vi "angulardistribution.vi"() -> ()   [LabVIEW 2024]
panel:
  out "THL":dbl
  out "2-14-25":i32
  out "1-13-25":i32
  out "23-11-25":i32
  out "12-24-25":i32
  in  "THL Discriminator 12":i32(slide) min=-250 max=0 step=5 scale=0.0..-250.0
  out "Seconds":i32
  out "10-22-25":i32
  out "9-21-25":i32
  out "8-20-25":i32
  out "7-19-25":i32
  out "6-18-25":i32
  out "5-17-25":i32
  out "4-16-25":i32
  out "3-15-25":i32
  in  "STOP":bool
  in  "START":bool
  in  "EXIT":bool
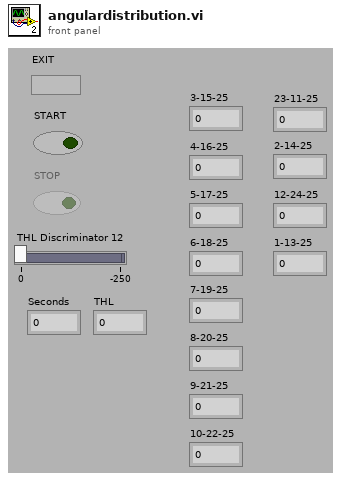
[diagram p1: front panel]
types:
  T1 = enum16{"Connect", "Set A", "Set B", "Set C", "Set D", "Set E", "Set F", "Set G", "Set H", "Get AND", "Read Counter", "Clear Counter"}
  T2 = enum16{"Connect", "Get IN", "Write Threshold", "Write Hysteresis", "Write Stretch"}
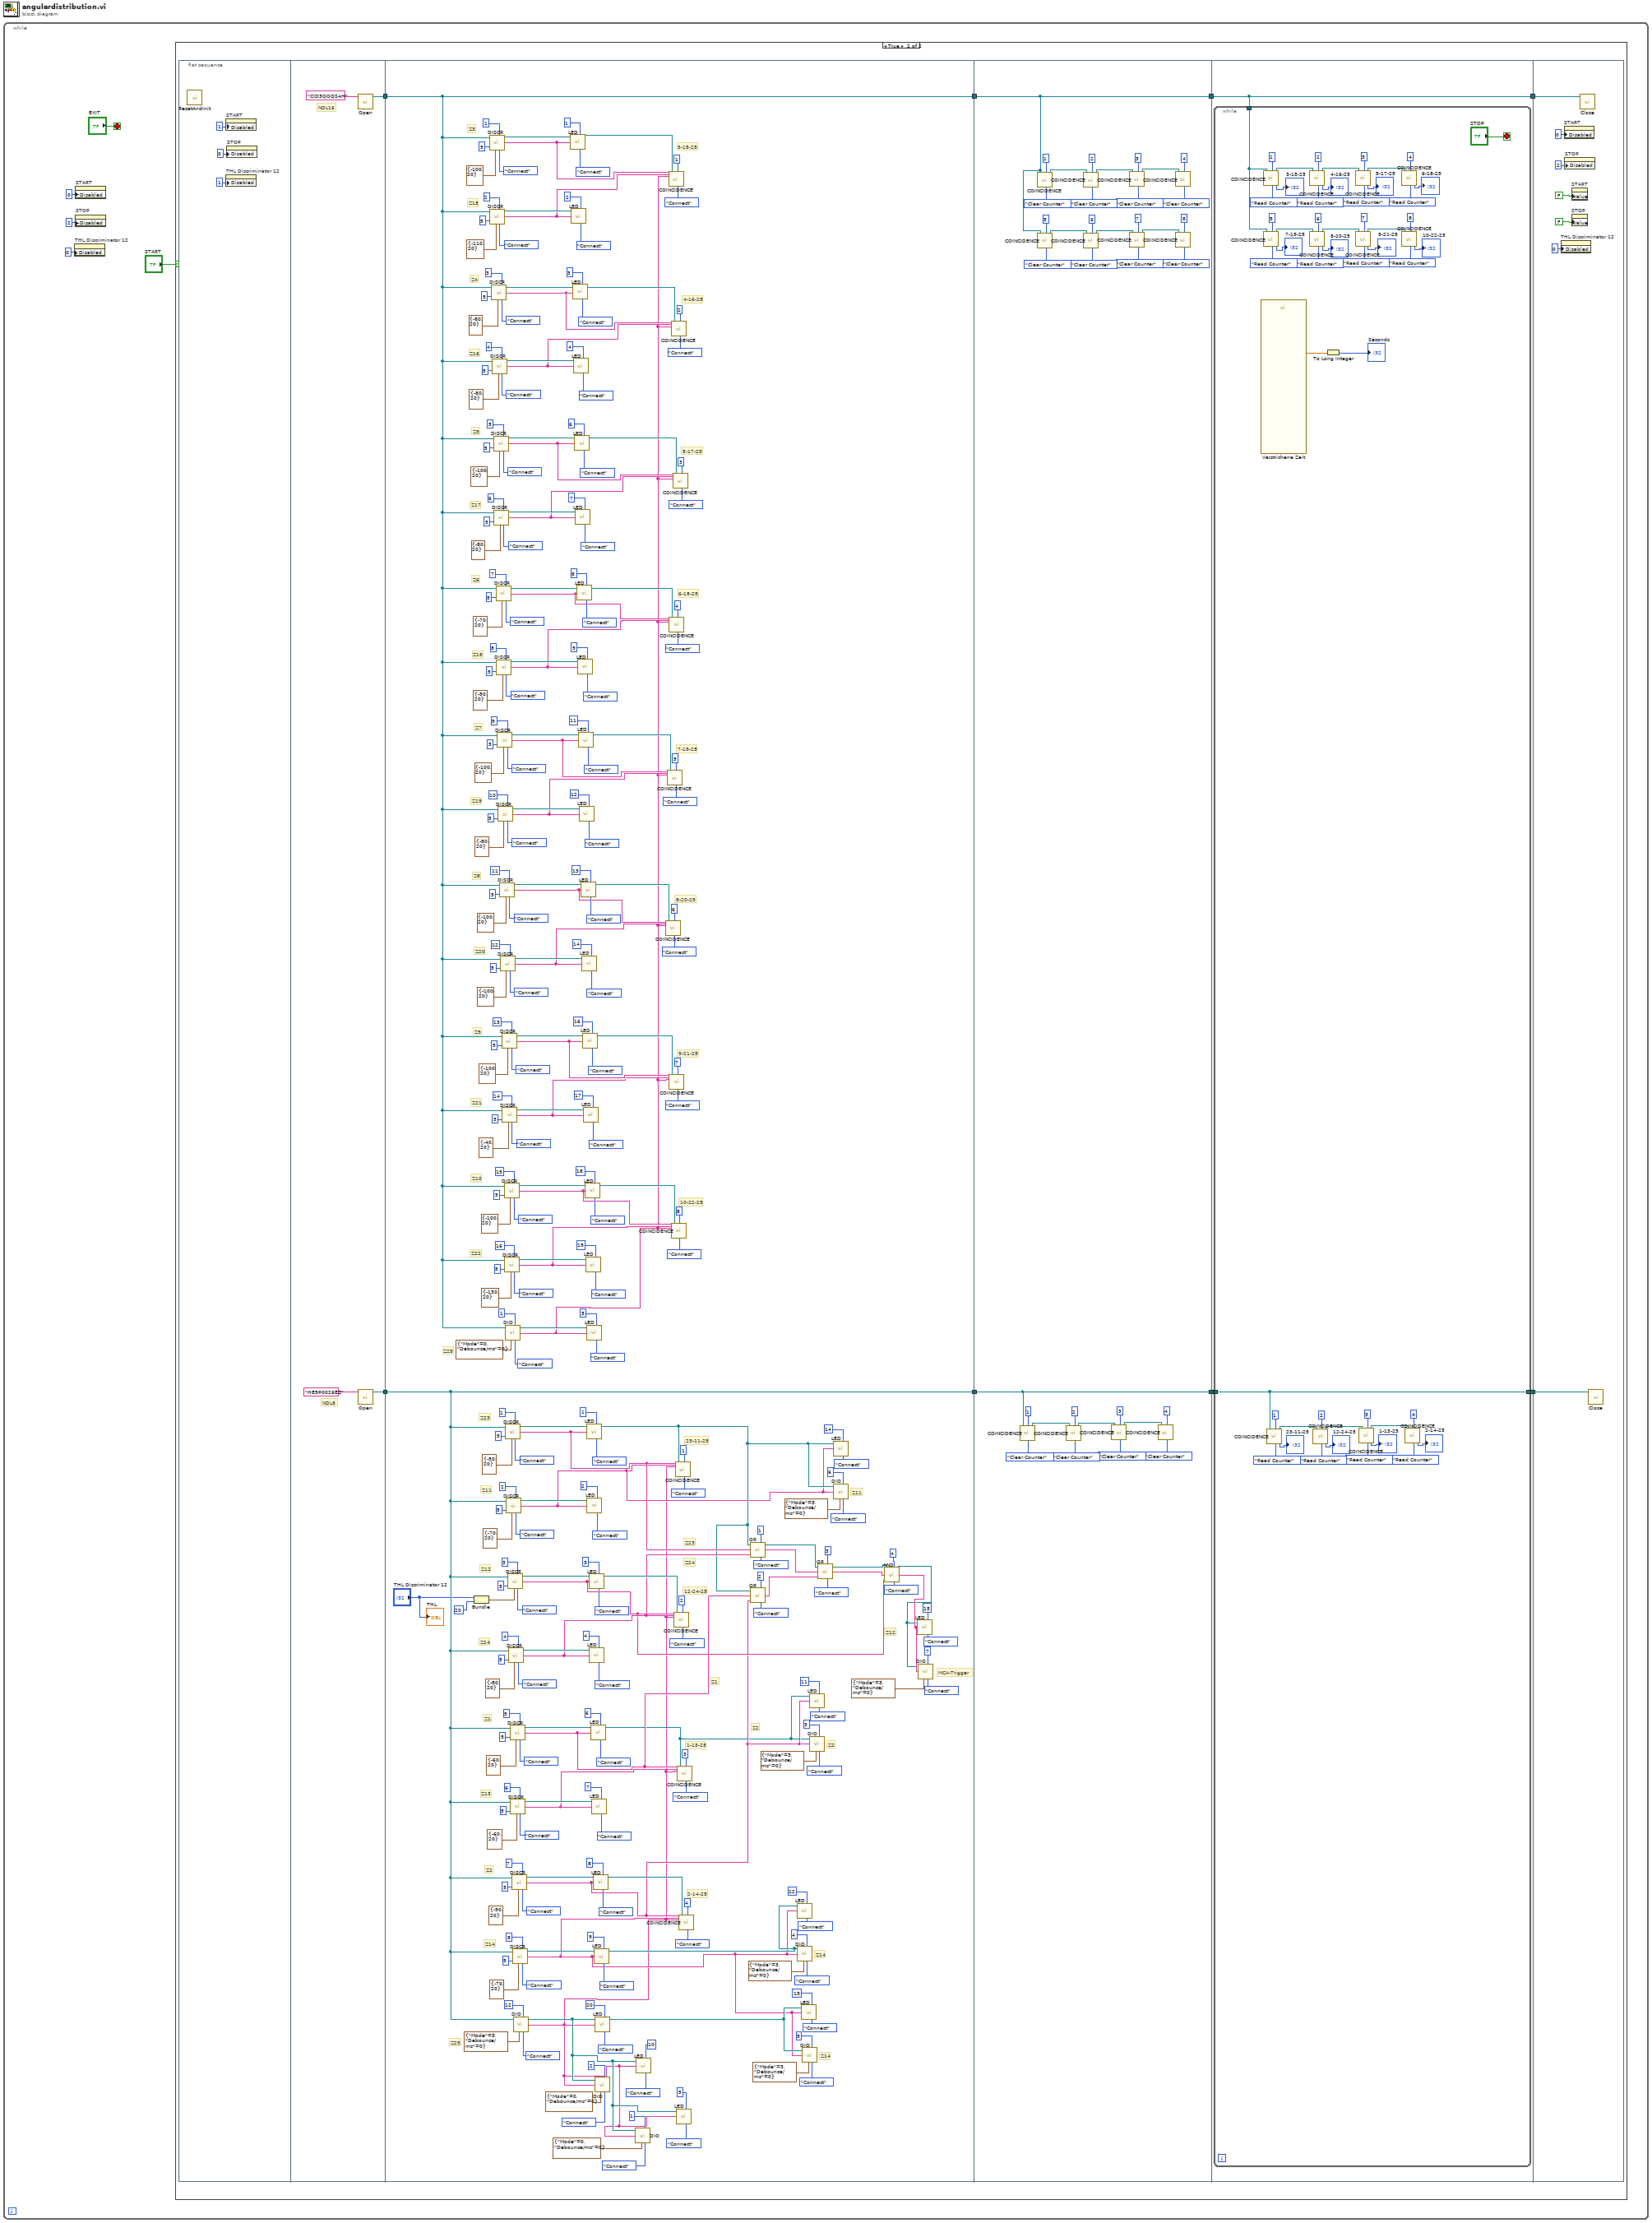
[diagram p0: block diagram]
diagram:
  n1 = while {
    stop <- "EXIT" stop-if-true
    n2 = property on="THL Discriminator 12" class="Schieber (strikt)"("Disabled"=u8 0 ("Deaktiviert")) -> ()  [unwired: 2 in, 2 out]
    n3 = property on="START" class="Bool. (strikt)"("Disabled"=u8 0 ("Deaktiviert")) -> ()  [unwired: 2 in, 2 out]
    n4 = property on="STOP" class="Bool. (strikt)"("Disabled"=u8 2 ("Deaktiviert")) -> ()  [unwired: 2 in, 2 out]
    n5 = case shown="True" "START" {
      frame False {
      }
      frame True {
        n6 = flat-sequence {
          tunnel: [w20] -> w13
          tunnel: [w17] -> w6
          tunnel: w13 -> [w31]
          tunnel: [w31] -> w12
          tunnel: [w92] -> w7
          tunnel: w6 -> [w92]
          tunnel: w12 -> [w331]
          tunnel: [w331] -> w11
          tunnel: [w319] -> w8
          tunnel: w7 -> [w319]
          tunnel: w11 -> [w356]
          tunnel: [w356] -> w10
          tunnel: [w355] -> w9
          tunnel: w8 -> [w354]
          tunnel: w10 -> [w411]
          tunnel: w9 -> [w407]
          frame #0 {
            n7 = call <userlib>:"ResetAndInit.vi"() -> ()  [unwired: 1 out]
            n8 = property on="START" class="Bool. (strikt)"("Disabled"=u8 1 ("Deaktiviert")) -> ()  [unwired: 2 in, 2 out]
            n9 = property on="THL Discriminator 12" class="Schieber (strikt)"("Disabled"=u8 1 ("Deaktiviert")) -> ()  [unwired: 2 in, 2 out]
            n10 = property on="STOP" class="Bool. (strikt)"("Disabled"=u8 0 ("Deaktiviert")) -> ()  [unwired: 2 in, 2 out]
          }
          frame #1 {
            # "NDL8"
            # "NDL16"
            n11 = call <userlib>:"Open.vi"("USB_LogicBox"="CID3QOQS4H") -> ("USB Out"=w20:refnum<visa-resource-name>)  [unwired: 1 in, 7 out]
            n12 = call <userlib>:"Open.vi"("USB_LogicBox"="HE5P0026EZ") -> ("USB Out"=w17:refnum<visa-resource-name>)  [unwired: 1 in, 7 out]
          }
          frame #2 {
            # "Z11"
            # "Z14"
            # "Z14"
            # "Z2"
            # "Z12"
            # "Z2"
            # "Z24"
            # "Z23"
            # "Z1"
            # "MCA-Trigger"
            # "2-14-25"
            # "1-13-25"
            # "12-24-25"
            # "23-11-25"
            # "Z25"
            # "Z14"
            # "Z2"
            # "Z13"
            # "Z1"
            # "Z24"
            # "Z12"
            # "Z11"
            # "Z23"
            # "10-22-25"
            # "9-21-25"
            # "8-20-25"
            # "7-19-25"
            # "6-18-25"
            # "5-17-25"
            # "4-16-25"
            # "3-15-25"
            # "Z25"
            # "Z22"
            # "Z10"
            # "Z21"
            # "Z9"
            # "Z20"
            # "Z8"
            # "Z19"
            # "Z7"
            # "Z18"
            # "Z6"
            # "Z17"
            # "Z5"
            # "Z16"
            # "Z4"
            # "Z15"
            # "Z3"
            n13 = Bundle("THL Discriminator 12"="THL Discriminator 12", 20) -> (w70:cluster{"THL Discriminator 12":i32, i32})  [unwired: 1 out]
            n14 = call <userlib>:"DISCR.vi"("USB In"=w31, "Stretch/10ns"=u8 5, "Params"=cluster{"Threshold/mV":i16, "Hysteresis/mV":u16} {"Threshold/mV"=-100, "Hysteresis/mV"=20}, "DISCR#"=u8 1, "Function"=T2."Connect") -> ("USB Out"=w314:refnum<visa-resource-name>, "DISCR"=w38:string)  [unwired: 3 out]
            n15 = call <userlib>:"DISCR.vi"("USB In"=w31, "Stretch/10ns"=u8 5, "Params"=cluster{"Threshold/mV":i16, "Hysteresis/mV":u16} {"Threshold/mV"=-110, "Hysteresis/mV"=20}, "DISCR#"=u8 2, "Function"=T2."Connect") -> ("USB Out"=w307:refnum<visa-resource-name>, "DISCR"=w37:string)  [unwired: 3 out]
            n16 = call <userlib>:"DISCR.vi"("USB In"=w31, "Stretch/10ns"=u8 5, "Params"=cluster{"Threshold/mV":i16, "Hysteresis/mV":u16} {"Threshold/mV"=-80, "Hysteresis/mV"=20}, "DISCR#"=u8 3, "Function"=T2."Connect") -> ("USB Out"=w300:refnum<visa-resource-name>, "DISCR"=w196:string)  [unwired: 3 out]
            n17 = call <userlib>:"DISCR.vi"("USB In"=w31, "Stretch/10ns"=u8 5, "Params"=cluster{"Threshold/mV":i16, "Hysteresis/mV":u16} {"Threshold/mV"=-80, "Hysteresis/mV"=20}, "DISCR#"=u8 4, "Function"=T2."Connect") -> ("USB Out"=w293:refnum<visa-resource-name>, "DISCR"=w194:string)  [unwired: 3 out]
            n18 = call <userlib>:"DISCR.vi"("USB In"=w31, "Stretch/10ns"=u8 5, "Params"=cluster{"Threshold/mV":i16, "Hysteresis/mV":u16} {"Threshold/mV"=-100, "Hysteresis/mV"=20}, "DISCR#"=u8 5, "Function"=T2."Connect") -> ("USB Out"=w286:refnum<visa-resource-name>, "DISCR"=w180:string)  [unwired: 3 out]
            n19 = call <userlib>:"DISCR.vi"("USB In"=w31, "Stretch/10ns"=u8 5, "Params"=cluster{"Threshold/mV":i16, "Hysteresis/mV":u16} {"Threshold/mV"=-80, "Hysteresis/mV"=20}, "DISCR#"=u8 6, "Function"=T2."Connect") -> ("USB Out"=w279:refnum<visa-resource-name>, "DISCR"=w179:string)  [unwired: 3 out]
            n20 = call <userlib>:"DISCR.vi"("USB In"=w31, "Stretch/10ns"=u8 5, "Params"=cluster{"Threshold/mV":i16, "Hysteresis/mV":u16} {"Threshold/mV"=-70, "Hysteresis/mV"=20}, "DISCR#"=u8 7, "Function"=T2."Connect") -> ("USB Out"=w272:refnum<visa-resource-name>, "DISCR"=w177:string)  [unwired: 3 out]
            n21 = call <userlib>:"DISCR.vi"("USB In"=w31, "Stretch/10ns"=u8 5, "Params"=cluster{"Threshold/mV":i16, "Hysteresis/mV":u16} {"Threshold/mV"=-50, "Hysteresis/mV"=20}, "DISCR#"=u8 8, "Function"=T2."Connect") -> ("USB Out"=w265:refnum<visa-resource-name>, "DISCR"=w176:string)  [unwired: 3 out]
            n22 = call <userlib>:"DISCR.vi"("USB In"=w31, "Stretch/10ns"=u8 5, "Params"=cluster{"Threshold/mV":i16, "Hysteresis/mV":u16} {"Threshold/mV"=-100, "Hysteresis/mV"=20}, "DISCR#"=u8 9, "Function"=T2."Connect") -> ("USB Out"=w258:refnum<visa-resource-name>, "DISCR"=w174:string)  [unwired: 3 out]
            n23 = call <userlib>:"DISCR.vi"("USB In"=w31, "Stretch/10ns"=u8 5, "Params"=cluster{"Threshold/mV":i16, "Hysteresis/mV":u16} {"Threshold/mV"=-80, "Hysteresis/mV"=20}, "DISCR#"=u8 10, "Function"=T2."Connect") -> ("USB Out"=w251:refnum<visa-resource-name>, "DISCR"=w173:string)  [unwired: 3 out]
            n24 = call <userlib>:"DISCR.vi"("USB In"=w31, "Stretch/10ns"=u8 5, "Params"=cluster{"Threshold/mV":i16, "Hysteresis/mV":u16} {"Threshold/mV"=-100, "Hysteresis/mV"=20}, "DISCR#"=u8 11, "Function"=T2."Connect") -> ("USB Out"=w244:refnum<visa-resource-name>, "DISCR"=w171:string)  [unwired: 3 out]
            n25 = call <userlib>:"DISCR.vi"("USB In"=w31, "Stretch/10ns"=u8 5, "Params"=cluster{"Threshold/mV":i16, "Hysteresis/mV":u16} {"Threshold/mV"=-100, "Hysteresis/mV"=20}, "DISCR#"=u8 12, "Function"=T2."Connect") -> ("USB Out"=w237:refnum<visa-resource-name>, "DISCR"=w170:string)  [unwired: 3 out]
            n26 = call <userlib>:"DISCR.vi"("USB In"=w31, "Stretch/10ns"=u8 5, "Params"=cluster{"Threshold/mV":i16, "Hysteresis/mV":u16} {"Threshold/mV"=-100, "Hysteresis/mV"=20}, "DISCR#"=u8 13, "Function"=T2."Connect") -> ("USB Out"=w230:refnum<visa-resource-name>, "DISCR"=w168:string)  [unwired: 3 out]
            n27 = call <userlib>:"DISCR.vi"("USB In"=w31, "Stretch/10ns"=u8 5, "Params"=cluster{"Threshold/mV":i16, "Hysteresis/mV":u16} {"Threshold/mV"=-40, "Hysteresis/mV"=20}, "DISCR#"=u8 14, "Function"=T2."Connect") -> ("USB Out"=w223:refnum<visa-resource-name>, "DISCR"=w167:string)  [unwired: 3 out]
            n28 = call <userlib>:"DISCR.vi"("USB In"=w31, "Stretch/10ns"=u8 5, "Params"=cluster{"Threshold/mV":i16, "Hysteresis/mV":u16} {"Threshold/mV"=-100, "Hysteresis/mV"=20}, "DISCR#"=u8 15, "Function"=T2."Connect") -> ("USB Out"=w216:refnum<visa-resource-name>, "DISCR"=w165:string)  [unwired: 3 out]
            n29 = call <userlib>:"DISCR.vi"("USB In"=w31, "Stretch/10ns"=u8 5, "Params"=cluster{"Threshold/mV":i16, "Hysteresis/mV":u16} {"Threshold/mV"=-130, "Hysteresis/mV"=20}, "DISCR#"=u8 16, "Function"=T2."Connect") -> ("USB Out"=w209:refnum<visa-resource-name>, "DISCR"=w164:string)  [unwired: 3 out]
            n30 = call <userlib>:"DIO.vi"("USB In"=w31, "Params"=cluster{"Mode":u8, "Debounce/ms":u8} {"Mode"=0, "Debounce/ms"=0}, "DIO#"=u8 1, "Function"=enum16{"Connect", "Set DO", "Get DI"}."Connect") -> ("USB Out"=w203:refnum<visa-resource-name>, "DI"=w29:string)  [unwired: 1 in, 3 out]
            n31 = call <userlib>:"DISCR.vi"("USB In"=w92, "Stretch/10ns"=u8 5, "Params"=cluster{"Threshold/mV":i16, "Hysteresis/mV":u16} {"Threshold/mV"=-50, "Hysteresis/mV"=20}, "DISCR#"=u8 1, "Function"=T2."Connect") -> ("USB Out"=w159:refnum<visa-resource-name>, "DISCR"=w87:string)  [unwired: 3 out]
            n32 = call <userlib>:"DISCR.vi"("USB In"=w92, "Stretch/10ns"=u8 5, "Params"=cluster{"Threshold/mV":i16, "Hysteresis/mV":u16} {"Threshold/mV"=-70, "Hysteresis/mV"=20}, "DISCR#"=u8 2, "Function"=T2."Connect") -> ("USB Out"=w152:refnum<visa-resource-name>, "DISCR"=w40:string)  [unwired: 3 out]
            n33 = call <userlib>:"DISCR.vi"("USB In"=w92, "Stretch/10ns"=u8 5, "Params"=w70, "DISCR#"=u8 3, "Function"=T2."Connect") -> ("USB Out"=w146:refnum<visa-resource-name>, "DISCR"=w76:string)  [unwired: 3 out]
            n34 = call <userlib>:"DISCR.vi"("USB In"=w92, "Stretch/10ns"=u8 5, "Params"=cluster{"Threshold/mV":i16, "Hysteresis/mV":u16} {"Threshold/mV"=-80, "Hysteresis/mV"=20}, "DISCR#"=u8 4, "Function"=T2."Connect") -> ("USB Out"=w139:refnum<visa-resource-name>, "DISCR"=w86:string)  [unwired: 3 out]
            n35 = call <userlib>:"DISCR.vi"("USB In"=w92, "Stretch/10ns"=u8 5, "Params"=cluster{"Threshold/mV":i16, "Hysteresis/mV":u16} {"Threshold/mV"=-60, "Hysteresis/mV"=20}, "DISCR#"=u8 5, "Function"=T2."Connect") -> ("USB Out"=w132:refnum<visa-resource-name>, "DISCR"=w85:string)  [unwired: 3 out]
            n36 = call <userlib>:"DISCR.vi"("USB In"=w92, "Stretch/10ns"=u8 5, "Params"=cluster{"Threshold/mV":i16, "Hysteresis/mV":u16} {"Threshold/mV"=-60, "Hysteresis/mV"=20}, "DISCR#"=u8 6, "Function"=T2."Connect") -> ("USB Out"=w125:refnum<visa-resource-name>, "DISCR"=w94:string)  [unwired: 3 out]
            n37 = call <userlib>:"DISCR.vi"("USB In"=w92, "Stretch/10ns"=u8 5, "Params"=cluster{"Threshold/mV":i16, "Hysteresis/mV":u16} {"Threshold/mV"=-90, "Hysteresis/mV"=20}, "DISCR#"=u8 7, "Function"=T2."Connect") -> ("USB Out"=w118:refnum<visa-resource-name>, "DISCR"=w63:string)  [unwired: 3 out]
            n38 = call <userlib>:"DISCR.vi"("USB In"=w92, "Stretch/10ns"=u8 5, "Params"=cluster{"Threshold/mV":i16, "Hysteresis/mV":u16} {"Threshold/mV"=-70, "Hysteresis/mV"=20}, "DISCR#"=u8 8, "Function"=T2."Connect") -> ("USB Out"=w111:refnum<visa-resource-name>, "DISCR"=w49:string)  [unwired: 3 out]
            n39 = call <userlib>:"DIO.vi"("USB In"=w92, "Params"=cluster{"Mode":u8, "Debounce/ms":u8} {"Mode"=3, "Debounce/ms"=0}, "DIO#"=u8 12, "Function"=enum16{"Connect", "Set DO", "Get DI"}."Connect") -> ("USB Out"=w25:refnum<visa-resource-name>, "DI"=w24:string)  [unwired: 1 in, 3 out]
            n40 = call <userlib>:"LED.vi"("USB In"=w314, "STATE"=w38, "LED#"=u8 1, "Function"=enum16{"Connect", "Set STATE"}."Connect") -> ("USB Out"=w30:refnum<visa-resource-name>)  [unwired: 5 out]
            n41 = call <userlib>:"LED.vi"("USB In"=w307, "STATE"=w37, "LED#"=u8 2, "Function"=enum16{"Connect", "Set STATE"}."Connect") -> ()  [unwired: 6 out]
            n42 = call <userlib>:"LED.vi"("USB In"=w300, "STATE"=w196, "LED#"=u8 3, "Function"=enum16{"Connect", "Set STATE"}."Connect") -> ("USB Out"=w195:refnum<visa-resource-name>)  [unwired: 5 out]
            n43 = call <userlib>:"LED.vi"("USB In"=w293, "STATE"=w194, "LED#"=u8 4, "Function"=enum16{"Connect", "Set STATE"}."Connect") -> ()  [unwired: 6 out]
            n44 = call <userlib>:"LED.vi"("USB In"=w286, "STATE"=w180, "LED#"=u8 6, "Function"=enum16{"Connect", "Set STATE"}."Connect") -> ("USB Out"=w181:refnum<visa-resource-name>)  [unwired: 5 out]
            n45 = call <userlib>:"LED.vi"("USB In"=w279, "STATE"=w179, "LED#"=u8 7, "Function"=enum16{"Connect", "Set STATE"}."Connect") -> ()  [unwired: 6 out]
            n46 = call <userlib>:"LED.vi"("USB In"=w272, "STATE"=w177, "LED#"=u8 8, "Function"=enum16{"Connect", "Set STATE"}."Connect") -> ("USB Out"=w178:refnum<visa-resource-name>)  [unwired: 5 out]
            n47 = call <userlib>:"LED.vi"("USB In"=w265, "STATE"=w176, "LED#"=u8 9, "Function"=enum16{"Connect", "Set STATE"}."Connect") -> ()  [unwired: 6 out]
            n48 = call <userlib>:"LED.vi"("USB In"=w258, "STATE"=w174, "LED#"=u8 11, "Function"=enum16{"Connect", "Set STATE"}."Connect") -> ("USB Out"=w175:refnum<visa-resource-name>)  [unwired: 5 out]
            n49 = call <userlib>:"LED.vi"("USB In"=w251, "STATE"=w173, "LED#"=u8 12, "Function"=enum16{"Connect", "Set STATE"}."Connect") -> ()  [unwired: 6 out]
            n50 = call <userlib>:"LED.vi"("USB In"=w244, "STATE"=w171, "LED#"=u8 13, "Function"=enum16{"Connect", "Set STATE"}."Connect") -> ("USB Out"=w172:refnum<visa-resource-name>)  [unwired: 5 out]
            n51 = call <userlib>:"LED.vi"("USB In"=w237, "STATE"=w170, "LED#"=u8 14, "Function"=enum16{"Connect", "Set STATE"}."Connect") -> ()  [unwired: 6 out]
            n52 = call <userlib>:"LED.vi"("USB In"=w230, "STATE"=w168, "LED#"=u8 16, "Function"=enum16{"Connect", "Set STATE"}."Connect") -> ("USB Out"=w169:refnum<visa-resource-name>)  [unwired: 5 out]
            n53 = call <userlib>:"LED.vi"("USB In"=w223, "STATE"=w167, "LED#"=u8 17, "Function"=enum16{"Connect", "Set STATE"}."Connect") -> ()  [unwired: 6 out]
            n54 = call <userlib>:"LED.vi"("USB In"=w216, "STATE"=w165, "LED#"=u8 18, "Function"=enum16{"Connect", "Set STATE"}."Connect") -> ("USB Out"=w166:refnum<visa-resource-name>)  [unwired: 5 out]
            n55 = call <userlib>:"LED.vi"("USB In"=w209, "STATE"=w164, "LED#"=u8 19, "Function"=enum16{"Connect", "Set STATE"}."Connect") -> ()  [unwired: 6 out]
            n56 = call <userlib>:"LED.vi"("USB In"=w203, "STATE"=w29, "LED#"=u8 5, "Function"=enum16{"Connect", "Set STATE"}."Connect") -> ()  [unwired: 6 out]
            n57 = call <userlib>:"LED.vi"("USB In"=w159, "STATE"=w87, "LED#"=u8 1, "Function"=enum16{"Connect", "Set STATE"}."Connect") -> ("USB Out"=w42:refnum<visa-resource-name>)  [unwired: 5 out]
            n58 = call <userlib>:"LED.vi"("USB In"=w152, "STATE"=w40, "LED#"=u8 2, "Function"=enum16{"Connect", "Set STATE"}."Connect") -> ()  [unwired: 6 out]
            n59 = call <userlib>:"LED.vi"("USB In"=w146, "STATE"=w76, "LED#"=u8 3, "Function"=enum16{"Connect", "Set STATE"}."Connect") -> ("USB Out"=w95:refnum<visa-resource-name>)  [unwired: 5 out]
            n60 = call <userlib>:"LED.vi"("USB In"=w139, "STATE"=w86, "LED#"=u8 4, "Function"=enum16{"Connect", "Set STATE"}."Connect") -> ()  [unwired: 6 out]
            n61 = call <userlib>:"LED.vi"("USB In"=w132, "STATE"=w85, "LED#"=u8 6, "Function"=enum16{"Connect", "Set STATE"}."Connect") -> ("USB Out"=w62:refnum<visa-resource-name>)  [unwired: 5 out]
            n62 = call <userlib>:"LED.vi"("USB In"=w125, "STATE"=w94, "LED#"=u8 7, "Function"=enum16{"Connect", "Set STATE"}."Connect") -> ()  [unwired: 6 out]
            n63 = call <userlib>:"LED.vi"("USB In"=w118, "STATE"=w63, "LED#"=u8 8, "Function"=enum16{"Connect", "Set STATE"}."Connect") -> ("USB Out"=w93:refnum<visa-resource-name>)  [unwired: 5 out]
            n64 = call <userlib>:"LED.vi"("USB In"=w111, "STATE"=w49, "LED#"=u8 9, "Function"=enum16{"Connect", "Set STATE"}."Connect") -> ("USB Out"=w56:refnum<visa-resource-name>)  [unwired: 5 out]
            n65 = call <userlib>:"LED.vi"("USB In"=w25, "STATE"=w24, "LED#"=u8 20, "Function"=enum16{"Connect", "Set STATE"}."Connect") -> ("USB Out"=w50:refnum<visa-resource-name>)  [unwired: 5 out]
            n66 = call <userlib>:"DIO.vi"("USB In"=w25, "DO"=w24, "Params"=cluster{"Mode":u8, "Debounce/ms":u8} {"Mode"=0, "Debounce/ms"=0}, "DIO#"=u8 2, "Function"=enum16{"Connect", "Set DO", "Get DI"}."Connect") -> ()  [unwired: 5 out]
            n67 = call <userlib>:"DIO.vi"("USB In"=w25, "DO"=w24, "Params"=cluster{"Mode":u8, "Debounce/ms":u8} {"Mode"=0, "Debounce/ms"=0}, "DIO#"=u8 1, "Function"=enum16{"Connect", "Set DO", "Get DI"}."Connect") -> ()  [unwired: 5 out]
            n68 = call <userlib>:"LED.vi"("USB In"=w25, "STATE"=w24, "LED#"=u8 10, "Function"=enum16{"Connect", "Set STATE"}."Connect") -> ()  [unwired: 6 out]
            n69 = call <userlib>:"COINCIDENCE.vi"("A"=w171, "B"=w170, "C"=w29, "USB In"=w172, "CC#"=u8 6, "Function"=T1."Connect") -> ()  [unwired: 5 in, 17 out]
            n70 = call <userlib>:"COINCIDENCE.vi"("A"=w174, "B"=w173, "C"=w29, "USB In"=w175, "CC#"=u8 5, "Function"=T1."Connect") -> ()  [unwired: 5 in, 17 out]
            n71 = call <userlib>:"COINCIDENCE.vi"("A"=w38, "B"=w37, "C"=w29, "USB In"=w30, "CC#"=u8 1, "Function"=T1."Connect") -> ()  [unwired: 5 in, 17 out]
            n72 = call <userlib>:"COINCIDENCE.vi"("A"=w177, "B"=w176, "C"=w29, "USB In"=w178, "CC#"=u8 4, "Function"=T1."Connect") -> ()  [unwired: 5 in, 17 out]
            n73 = call <userlib>:"COINCIDENCE.vi"("A"=w168, "B"=w167, "C"=w29, "USB In"=w169, "CC#"=u8 7, "Function"=T1."Connect") -> ()  [unwired: 5 in, 17 out]
            n74 = call <userlib>:"COINCIDENCE.vi"("A"=w165, "B"=w164, "C"=w29, "USB In"=w166, "CC#"=u8 8, "Function"=T1."Connect") -> ()  [unwired: 5 in, 17 out]
            n75 = call <userlib>:"COINCIDENCE.vi"("A"=w196, "B"=w194, "C"=w29, "USB In"=w195, "CC#"=u8 2, "Function"=T1."Connect") -> ()  [unwired: 5 in, 17 out]
            n76 = call <userlib>:"COINCIDENCE.vi"("A"=w180, "B"=w179, "C"=w29, "USB In"=w181, "CC#"=u8 3, "Function"=T1."Connect") -> ()  [unwired: 5 in, 17 out]
            n77 = call <userlib>:"COINCIDENCE.vi"("A"=w76, "B"=w86, "C"=w24, "USB In"=w95, "CC#"=u8 2, "Function"=T1."Connect") -> ()  [unwired: 5 in, 17 out]
            n78 = call <userlib>:"COINCIDENCE.vi"("A"=w87, "B"=w40, "C"=w24, "USB In"=w42, "CC#"=u8 1, "Function"=T1."Connect") -> ()  [unwired: 5 in, 17 out]
            n79 = call <userlib>:"LED.vi"("USB In"=w25, "STATE"=w24, "LED#"=u8 5, "Function"=enum16{"Connect", "Set STATE"}."Connect") -> ()  [unwired: 6 out]
            n80 = call <userlib>:"COINCIDENCE.vi"("A"=w85, "B"=w94, "C"=w24, "USB In"=w62, "CC#"=u8 3, "Function"=T1."Connect") -> ()  [unwired: 5 in, 17 out]
            n81 = call <userlib>:"COINCIDENCE.vi"("A"=w63, "B"=w49, "C"=w24, "USB In"=w93, "CC#"=u8 4, "Function"=T1."Connect") -> ()  [unwired: 5 in, 17 out]
            n82 = call <userlib>:"OR.vi"("USB In"=w42, "A"=w87, "B"=w86, "LOGIC#"=u8 1, "Function"=enum16{"Connect", "Set A", "Set B", "Get OR"}."Connect") -> ("USB Out"=w83:refnum<visa-resource-name>, "OR"=w82:string)  [unwired: 3 out]
            n83 = call <userlib>:"OR.vi"("USB In"=w42, "A"=w85, "B"=w63, "LOGIC#"=u8 2, "Function"=enum16{"Connect", "Set A", "Set B", "Get OR"}."Connect") -> ("OR"=w81:string)  [unwired: 4 out]
            n84 = call <userlib>:"LED.vi"("USB In"=w56, "STATE"=w49, "LED#"=u8 12, "Function"=enum16{"Connect", "Set STATE"}."Connect") -> ()  [unwired: 6 out]
            n85 = call <userlib>:"DIO.vi"("USB In"=w56, "DO"=w49, "Params"=cluster{"Mode":u8, "Debounce/ms":u8} {"Mode"=3, "Debounce/ms"=0}, "DIO#"=u8 4, "Function"=enum16{"Connect", "Set DO", "Get DI"}."Connect") -> ()  [unwired: 5 out]
            n86 = call <userlib>:"LED.vi"("USB In"=w50, "STATE"=w49, "LED#"=u8 13, "Function"=enum16{"Connect", "Set STATE"}."Connect") -> ()  [unwired: 6 out]
            n87 = call <userlib>:"DIO.vi"("USB In"=w50, "DO"=w49, "Params"=cluster{"Mode":u8, "Debounce/ms":u8} {"Mode"=3, "Debounce/ms"=0}, "DIO#"=u8 5, "Function"=enum16{"Connect", "Set DO", "Get DI"}."Connect") -> ()  [unwired: 5 out]
            n88 = call <userlib>:"LED.vi"("USB In"=w62, "STATE"=w63, "LED#"=u8 11, "Function"=enum16{"Connect", "Set STATE"}."Connect") -> ()  [unwired: 6 out]
            n89 = call <userlib>:"DIO.vi"("USB In"=w62, "DO"=w63, "Params"=cluster{"Mode":u8, "Debounce/ms":u8} {"Mode"=3, "Debounce/ms"=0}, "DIO#"=u8 3, "Function"=enum16{"Connect", "Set DO", "Get DI"}."Connect") -> ()  [unwired: 5 out]
            n90 = call <userlib>:"OR.vi"("USB In"=w83, "A"=w82, "B"=w81, "LOGIC#"=u8 3, "Function"=enum16{"Connect", "Set A", "Set B", "Get OR"}."Connect") -> ("USB Out"=w78:refnum<visa-resource-name>, "OR"=w77:string)  [unwired: 3 out]
            n91 = call <userlib>:"LED.vi"("USB In"=w42, "STATE"=w40, "LED#"=u8 14, "Function"=enum16{"Connect", "Set STATE"}."Connect") -> ()  [unwired: 6 out]
            n92 = call <userlib>:"DIO.vi"("USB In"=w42, "DO"=w40, "Params"=cluster{"Mode":u8, "Debounce/ms":u8} {"Mode"=3, "Debounce/ms"=0}, "DIO#"=u8 6, "Function"=enum16{"Connect", "Set DO", "Get DI"}."Connect") -> ()  [unwired: 5 out]
            n93 = call <userlib>:"AND.vi"("USB In"=w78, "A"=w77, "B"=w76, "LOGIC#"=u8 4 ("CC#"), "Function"=enum16{"Connect", "Set A", "Set B", "Get AND"}."Connect") -> ("USB Out"=w43:refnum<visa-resource-name>, "AND"=w44:string)  [unwired: 3 out]
            n94 = call <userlib>:"LED.vi"("USB In"=w43, "STATE"=w44, "LED#"=u8 15, "Function"=enum16{"Connect", "Set STATE"}."Connect") -> ()  [unwired: 6 out]
            n95 = call <userlib>:"DIO.vi"("USB In"=w43, "DO"=w44, "Params"=cluster{"Mode":u8, "Debounce/ms":u8} {"Mode"=3, "Debounce/ms"=0}, "DIO#"=u8 7, "Function"=enum16{"Connect", "Set DO", "Get DI"}."Connect") -> ()  [unwired: 5 out]
            "THL" <- "THL Discriminator 12"
          }
          frame #3 {
            n96 = call <userlib>:"COINCIDENCE.vi"("USB In"=w319, "CC#"=u8 1, "Function"=T1."Clear Counter") -> ("USB Out"=w322:refnum<visa-resource-name>)  [unwired: 8 in, 16 out]
            n97 = call <userlib>:"COINCIDENCE.vi"("USB In"=w331, "CC#"=u8 1, "Function"=T1."Clear Counter") -> ("USB Out"=w345:refnum<visa-resource-name>)  [unwired: 8 in, 16 out]
            n98 = call <userlib>:"COINCIDENCE.vi"("USB In"=w331, "CC#"=u8 5, "Function"=T1."Clear Counter") -> ("USB Out"=w334:refnum<visa-resource-name>)  [unwired: 8 in, 16 out]
            n99 = call <userlib>:"COINCIDENCE.vi"("USB In"=w322, "CC#"=u8 2, "Function"=T1."Clear Counter") -> ("USB Out"=w321:refnum<visa-resource-name>)  [unwired: 8 in, 16 out]
            n100 = call <userlib>:"COINCIDENCE.vi"("USB In"=w345, "CC#"=u8 2, "Function"=T1."Clear Counter") -> ("USB Out"=w344:refnum<visa-resource-name>)  [unwired: 8 in, 16 out]
            n101 = call <userlib>:"COINCIDENCE.vi"("USB In"=w334, "CC#"=u8 6, "Function"=T1."Clear Counter") -> ("USB Out"=w333:refnum<visa-resource-name>)  [unwired: 8 in, 16 out]
            n102 = call <userlib>:"COINCIDENCE.vi"("USB In"=w321, "CC#"=u8 3, "Function"=T1."Clear Counter") -> ("USB Out"=w320:refnum<visa-resource-name>)  [unwired: 8 in, 16 out]
            n103 = call <userlib>:"COINCIDENCE.vi"("USB In"=w344, "CC#"=u8 3, "Function"=T1."Clear Counter") -> ("USB Out"=w343:refnum<visa-resource-name>)  [unwired: 8 in, 16 out]
            n104 = call <userlib>:"COINCIDENCE.vi"("USB In"=w333, "CC#"=u8 7, "Function"=T1."Clear Counter") -> ("USB Out"=w332:refnum<visa-resource-name>)  [unwired: 8 in, 16 out]
            n105 = call <userlib>:"COINCIDENCE.vi"("USB In"=w320, "CC#"=u8 4, "Function"=T1."Clear Counter") -> ()  [unwired: 8 in, 17 out]
            n106 = call <userlib>:"COINCIDENCE.vi"("USB In"=w343, "CC#"=u8 4, "Function"=T1."Clear Counter") -> ()  [unwired: 8 in, 17 out]
            n107 = call <userlib>:"COINCIDENCE.vi"("USB In"=w332, "CC#"=u8 8, "Function"=T1."Clear Counter") -> ()  [unwired: 8 in, 17 out]
          }
          frame #4 {
            n108 = while {
              tunnel: w356 -> [w383]
              tunnel: [w361] -> w355
              tunnel: w354 -> [w361]
              stop <- "STOP" stop-if-true
              n109 = call "Verstrichene Zeit"() -> ("Elapsed Time (s)"=w374:dbl)  [unwired: 5 in, 14 out]
              n110 = call <userlib>:"COINCIDENCE.vi"("USB In"=w383, "CC#"=u8 1, "Function"=T1."Read Counter") -> ("USB Out"=w392:refnum<visa-resource-name>, "Counter"=→"3-15-25":u32)  [unwired: 8 in, 15 out]
              n111 = call <userlib>:"COINCIDENCE.vi"("USB In"=w383, "CC#"=u8 5, "Function"=T1."Read Counter") -> ("USB Out"=w403:refnum<visa-resource-name>, "Counter"=→"7-19-25":u32)  [unwired: 8 in, 15 out]
              n112 = call <userlib>:"COINCIDENCE.vi"("USB In"=w361, "CC#"=u8 1, "Function"=T1."Read Counter") -> ("USB Out"=w364:refnum<visa-resource-name>, "Counter"=→"23-11-25":u32)  [unwired: 8 in, 15 out]
              n113 = call <userlib>:"COINCIDENCE.vi"("USB In"=w392, "CC#"=u8 2, "Function"=T1."Read Counter") -> ("USB Out"=w393:refnum<visa-resource-name>, "Counter"=→"4-16-25":u32)  [unwired: 8 in, 15 out]
              n114 = call <userlib>:"COINCIDENCE.vi"("USB In"=w403, "CC#"=u8 6, "Function"=T1."Read Counter") -> ("USB Out"=w404:refnum<visa-resource-name>, "Counter"=→"8-20-25":u32)  [unwired: 8 in, 15 out]
              n115 = call <userlib>:"COINCIDENCE.vi"("USB In"=w364, "CC#"=u8 2, "Function"=T1."Read Counter") -> ("USB Out"=w363:refnum<visa-resource-name>, "Counter"=→"12-24-25":u32)  [unwired: 8 in, 15 out]
              n116 = To Long Integer(number=w374) -> (32bit integer=→"Seconds":i32)
              n117 = call <userlib>:"COINCIDENCE.vi"("USB In"=w393, "CC#"=u8 3, "Function"=T1."Read Counter") -> ("USB Out"=w394:refnum<visa-resource-name>, "Counter"=→"5-17-25":u32)  [unwired: 8 in, 15 out]
              n118 = call <userlib>:"COINCIDENCE.vi"("USB In"=w404, "CC#"=u8 7, "Function"=T1."Read Counter") -> ("USB Out"=w405:refnum<visa-resource-name>, "Counter"=→"9-21-25":u32)  [unwired: 8 in, 15 out]
              n119 = call <userlib>:"COINCIDENCE.vi"("USB In"=w363, "CC#"=u8 3, "Function"=T1."Read Counter") -> ("USB Out"=w362:refnum<visa-resource-name>, "Counter"=→"1-13-25":u32)  [unwired: 8 in, 15 out]
              n120 = call <userlib>:"COINCIDENCE.vi"("USB In"=w394, "CC#"=u8 4, "Function"=T1."Read Counter") -> ("Counter"=→"6-18-25":u32)  [unwired: 8 in, 16 out]
              n121 = call <userlib>:"COINCIDENCE.vi"("USB In"=w405, "CC#"=u8 8, "Function"=T1."Read Counter") -> ("Counter"=→"10-22-25":u32)  [unwired: 8 in, 16 out]
              n122 = call <userlib>:"COINCIDENCE.vi"("USB In"=w362, "CC#"=u8 4, "Function"=T1."Read Counter") -> ("Counter"=→"2-14-25":u32)  [unwired: 8 in, 16 out]
            }
          }
          frame #5 {
            n123 = property on="THL Discriminator 12" class="Schieber (strikt)"("Disabled"=u8 0 ("Deaktiviert")) -> ()  [unwired: 2 in, 2 out]
            n124 = property on="START" class="Bool. (strikt)"("Disabled"=u8 0 ("Deaktiviert")) -> ()  [unwired: 2 in, 2 out]
            n125 = property on="STOP" class="Bool. (strikt)"("Disabled"=u8 2 ("Deaktiviert")) -> ()  [unwired: 2 in, 2 out]
            n126 = property on="START" class="Bool. (strikt)"("Value"=FALSE ("START")) -> ()  [unwired: 2 in, 2 out]
            n127 = property on="STOP" class="Bool. (strikt)"("Value"=FALSE ("STOP")) -> ()  [unwired: 2 in, 2 out]
            n128 = call <userlib>:"Close.vi"("USB In"=w411) -> ()  [unwired: 1 in, 8 out]
            n129 = call <userlib>:"Close.vi"("USB In"=w407) -> ()  [unwired: 1 in, 8 out]
          }
        }
      }
    }
  }
